vi "Available Staffs.vi"(0 "Incoming Hotel Management Tool Model Interface in":refnum<class "Incoming Hotel Management Tool Model Interface.lvclass">, 5 "Staff Name":string[](array[string]), 11 "error in (no error)":errorcluster) -> (4 "Incoming Hotel Management Tool Model Interface out":refnum<class "Incoming Hotel Management Tool Model Interface.lvclass">, 15 "error out":errorcluster)   [LabVIEW 2023, in "Incoming Hotel Management Tool Model Interface.lvlib" / "Incoming Hotel Management Tool Model Interface.lvclass"]
uses:
  Incoming Hotel Management Tool Model Interface.lvclass
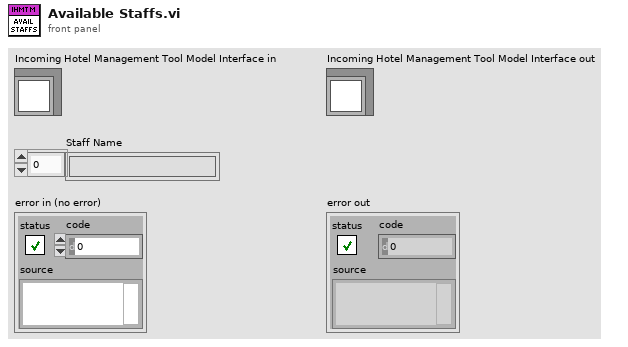
[diagram p1: front panel]
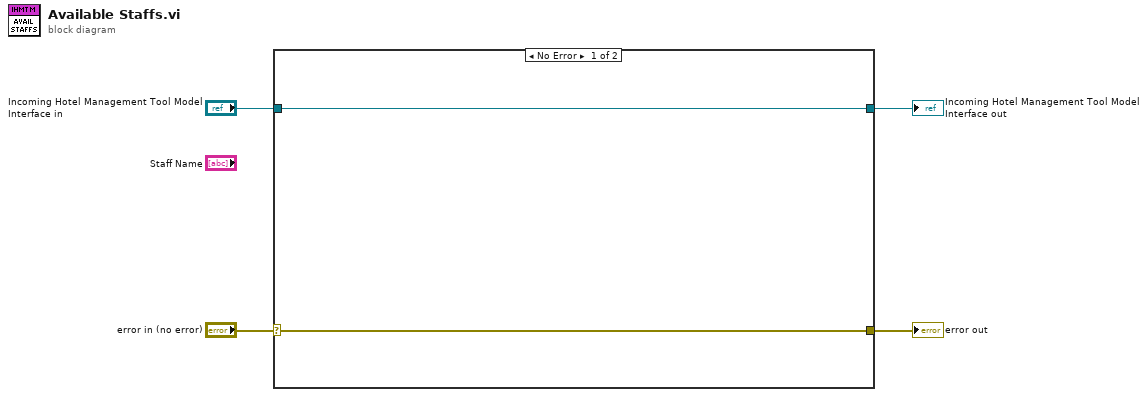
[diagram p0: block diagram]
diagram:
  n1 = case shown="No Error" "error in (no error)" {
    selector: "error in (no error)" -> [w5 w8]
    tunnel: [w5 w8] -> w3
    tunnel: [w6 w7] -> w1
    tunnel: "Incoming Hotel Management Tool Model Interface in" -> [w6 w7]
    frame No Error {
    }
    frame Error {
    }
  }
  "error out" <- w3
  "Incoming Hotel Management Tool Model Interface out" <- w1
